vi "dbTest.vi"() -> ()   [LabVIEW 2015]
uses:
  C:/Users/Arkadiusz/SkyDrive/Dokumenty/Visual Studio 2015/Projects/NordicDatabaseDLL/NordicDatabaseDLL/bin/Debug/NordicDatabaseDLL.dll
  Visual Studio 2015/Projects/NordicDatabaseDLL/NordicDatabaseDLL/bin/Debug/NordicDatabaseDLL.dll
panel:
  in  "Boolean":bool
  in  "stop":bool
  out "SelectDataTemperature":sgl[](array[numeric])
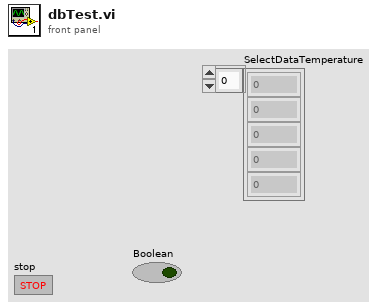
[diagram p1: front panel]
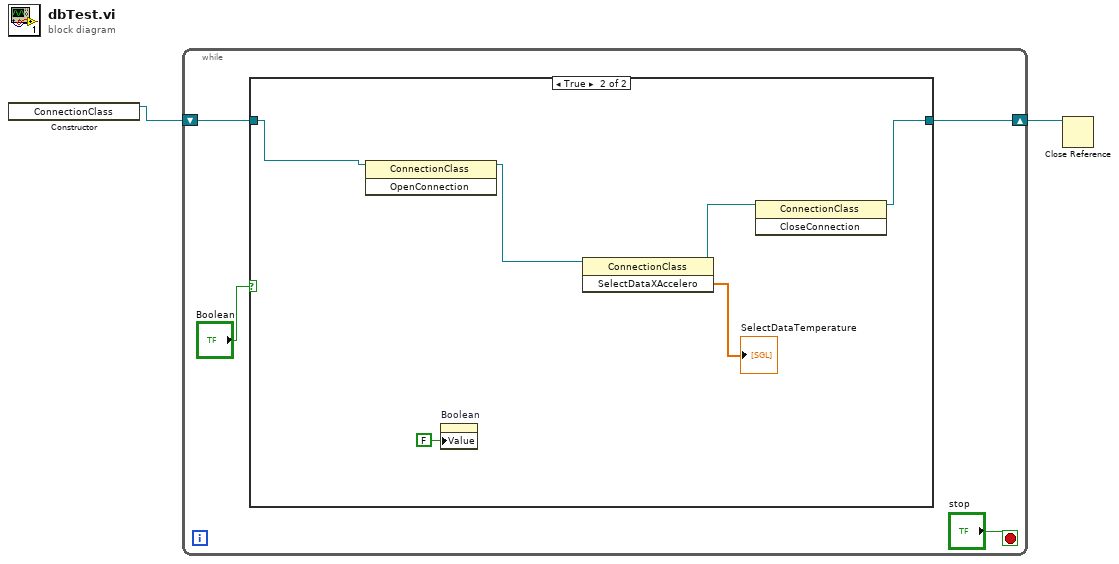
[diagram p0: block diagram]
diagram:
  n1 = constructor class="ConnectionClass"() -> (reference out=w2:refnum<k24>)  [unwired: 3 in, 2 out]
  n2 = while {
    shift-right: [w3] -> w1
    shift-left: w2 -> [w6]
    stop <- "stop" stop-if-true
    n3 = case shown="True" "Boolean" {
      tunnel: w6 -> [w7 w9]
      tunnel: [w7 w11] -> w3
      frame False {
      }
      frame True {
        n4 = invoke class="ConnectionClass" method="OpenConnection"(reference=w9) -> (reference out=w8:refnum<k24>)  [unwired: 2 in, 2 out]
        n5 = property on="Boolean" class="Bool (strict)"("Value"=FALSE ("Boolean")) -> ()  [unwired: 2 in, 2 out]
        n6 = invoke class="ConnectionClass" method="SelectDataXAccelero"(reference=w8) -> (reference out=w12:refnum<k24>, "SelectDataXAccelero"=→"SelectDataTemperature":sgl[])  [unwired: 2 in, 1 out]
        n7 = invoke class="ConnectionClass" method="CloseConnection"(reference=w12) -> (reference out=w11:refnum<k24>)  [unwired: 2 in, 2 out]
      }
    }
  }
  n8 = Close Reference(reference=w1) -> ()  [unwired: 1 in, 1 out]
